vi "Diagnostic Unlock ECU Service.vi"(10 "NIVS.Workspace Event":refnum<event-registration>, 11 "NIVS.Gateway IP Address":string="localhost") -> ()   [LabVIEW 2024, in "Diagnostic Unlock ECU Service.lvlib"]
uses:
  Diagnostic Unlock ECU Service.lvlib
  Types/State Variables.ctl
  <vilib>/NI VeriStand/Execution/Workspace/WorkspaceAPI.ctl
  <vilib>/Platform/TimedLoop/XDataNode/timing_clust.ctl
  <vilib>/Platform/TimedLoop/XDataNode/nitl_modes.ctl
  <vilib>/Platform/TimedLoop/XDataNode/wakeup.ctl
  <vilib>/Utility/error.llb/DialogType.ctl
  <vilib>/Platform/TimedLoop/XDataNode/XDataNode.xnode
  <vilib>/NI VeriStand/Execution/Workspace/NI_VS Workspace ExecutionAPI.lvlib
  <vilib>/Platform/TimedLoop/XDataNode/XDNodeRunTimeDep.lvlib
  <vilib>/Utility/SystemLogging/NI_SystemLogging.lvlib
  NationalInstruments.VeriStand.ClientAPI
panel:
  in  "Stop":bool
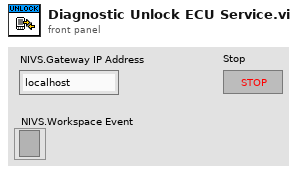
[diagram p1: front panel]
types:
  T1 = typedef "Diagnostic Unlock ECU Service.lvlib/State Variables.ctl" = cluster{"VS.Workspace.Ref":T2, "VS.Connected?":bool, "TCP.Listener":refnum<k5>, "Name":string}
  T2 = typedef "NI_VS Workspace ExecutionAPI.lvlib/WorkspaceAPI.ctl" = refnum<k24>
  T3 = typedef "NI_VS Workspace ExecutionAPI.lvlib/SystemStateEventRef.ctl" = cluster{"CustDatRef":refnum<user-event>, "EvtRef":refnum<k27>, "Target State User Event":refnum<user-event>}
  T4 = typedef "NI_VS Workspace ExecutionAPI.lvlib/SystemStateRegEventRef.ctl" = refnum<event-registration>
  T5 = cluster{"NIVS.Workspace Event":refnum<event-registration>, "SystemChangeEventRef":T4}
  T6 = typedef "XDNodeRunTimeDep.lvlib/timing_clust.ctl" = cluster{"Expected End [f-1]":u64, "Actual End [f-1]":u64, "Finished Late? [f-1]":bool, "Expected End [i-1]":u64, "Actual End [i-1]":u64, "Finished Late? [i-1]":bool, "Expected Start [i]":u64, "Actual Start [i]":u64, "Expected Start [f]":u64, "Actual Start [f]":u64, "Source Name":string, "Structure Name":string, "Period":i64, "Deadline":i64, "Offset":i64, "Start":i64, "Priority":i32, "Timeout":i32, "Mode":T7, "Wakeup Reason":T8, "Error":errorcluster, "Source Type":string, "Secondary Source Type":string, "Global End Time":u64, "Global Start Time":u64, "Frame Duration":u64, "Iteration Duration":u64, "Assigned CPU":i32, "I/O Scan Engine Mode":u32}
  T7 = typedef "XDNodeRunTimeDep.lvlib/nitl_modes.ctl" = enum32{"No Change", "Process missed periods, maintain original phase", "Discard missed periods, maintain original phase", "Process missed periods, ignore original phase", "Discard missed periods, ignore original phase"}
  T8 = typedef "XDNodeRunTimeDep.lvlib/wakeup.ctl" = enum32{"Normal", "Aborted", "Asynchronous wakeup", "Timing source error", "Timed loop error", "Timeout"}
  T9 = typedef "NI_VS Workspace ExecutionAPI.lvlib/SystemState.ctl" = u8
  T10 = typedef "DialogType.ctl" = u16
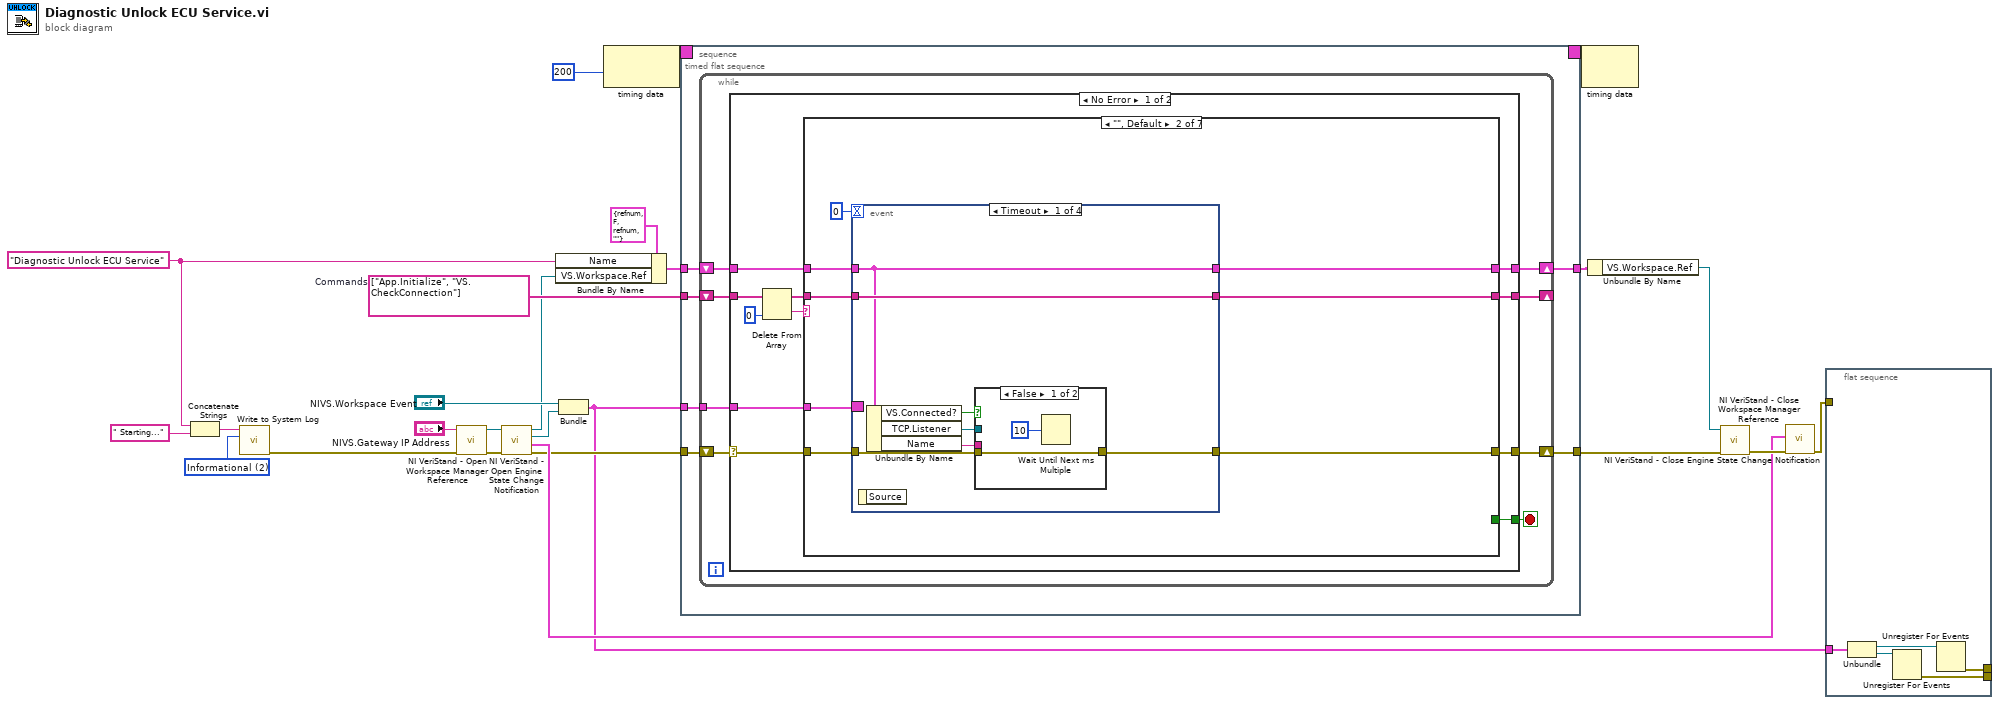
[diagram p0: block diagram]
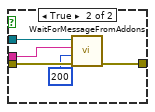
[diagram p3: hidden frame]
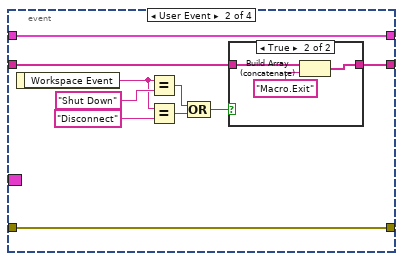
[diagram p4: hidden frame]
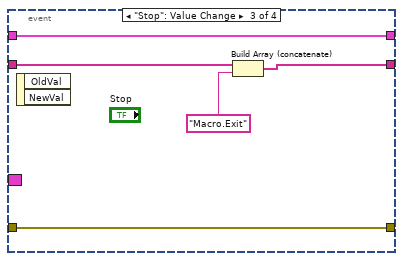
[diagram p6: hidden frame]
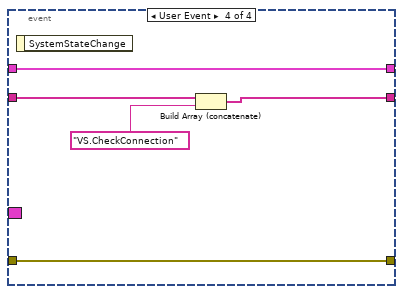
[diagram p7: hidden frame]
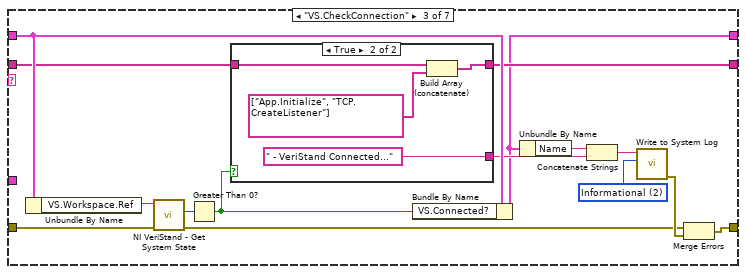
[diagram p8: hidden frame]
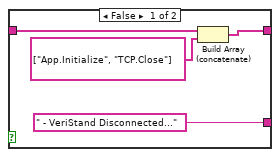
[diagram p9: hidden frame]
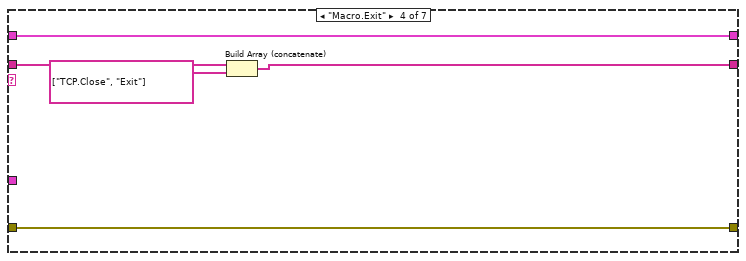
[diagram p10: hidden frame]
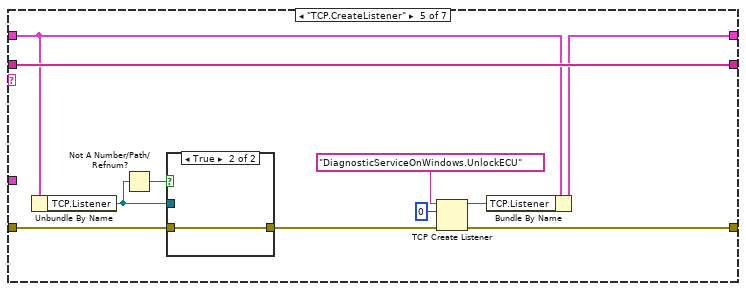
[diagram p11: hidden frame]
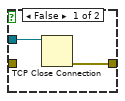
[diagram p12: hidden frame]
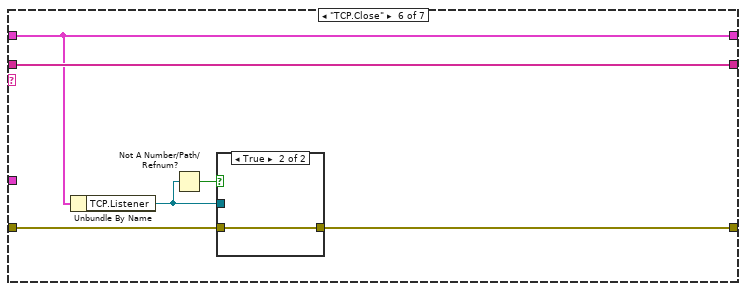
[diagram p13: hidden frame]
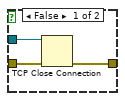
[diagram p14: hidden frame]
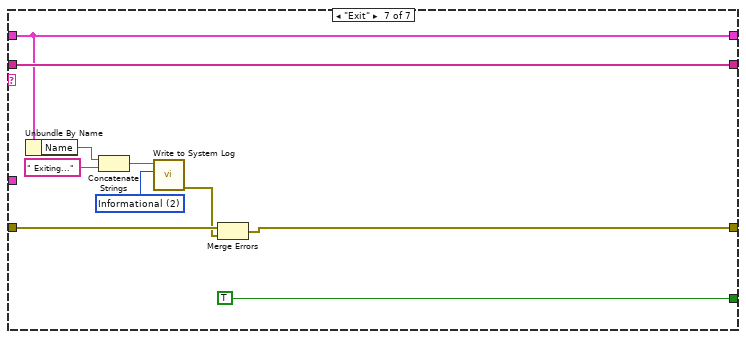
[diagram p15: hidden frame]
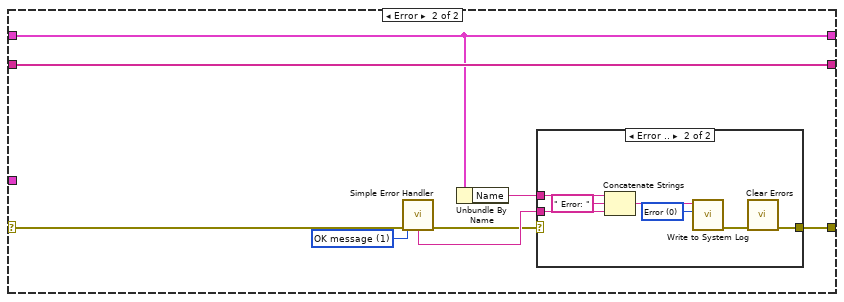
[diagram p16: hidden frame]
diagram:
  w1 = "Diagnostic Unlock ECU Service" ("string")
  w8 = 2 items=["Error", "Warning", "Informational"] ("severity")
  w19 = string[] ["App.Initialize", "VS.CheckConnection"]  # Commands
  n1 = Concatenate Strings(w1, " Starting..." ("message")) -> (w3:string)
  n2 = call <vilib>:"Write to System Log.vi"("severity"=w8, "message"=w3) -> ("error out"=w7:errorcluster)  [unwired: 9 in]
  n3 = call <vilib>:"NI VeriStand - Open Workspace Manager Reference.vi"("error in (no error)"=w7, "Gateway IP Address (\"\": localhost)"="NIVS.Gateway IP Address") -> ("error out"=w5:errorcluster, "WorkspaceManager"=w25:T2)  [unwired: 8 in]
  n4 = call <vilib>:"NI VeriStand - Open Engine State Change Notification.vi"("error in (no error)"=w5, "WorkspaceManager in"=w25) -> ("error out"=w20:errorcluster, "SystemStateRefs"=w23:T3, "SystemChangeEventRef"=w21:T4, "WorkspaceManager out"=w16:T2)  [unwired: 6 in]
  n5 = Bundle By Name(cluster=T1 {"VS.Workspace.Ref"=refnum, "VS.Connected?"=FALSE, "TCP.Listener"=refnum, "Name"=""}, "Name"=w1, "VS.Workspace.Ref"=w16) -> (w14:T1)
  n6 = Bundle("NIVS.Workspace Event"="NIVS.Workspace Event", "SystemChangeEventRef"=w21) -> (w18:T5)  [unwired: 1 in]
  n7 = node-c288(200 ("Priority")) -> (w11:T6)
  n8 = timed-sequence {
    timing: w11 -> [_]
    timing-out: [_] -> w10
    tunnel: [w31] -> w4
    tunnel: w20 -> [w30]
    tunnel: w19 -> [w29]
    tunnel: w18 -> [w28]
    tunnel: w14 -> [w27]
    tunnel: [w26] -> w13
    n9 = timed-flat-sequence {
      tunnel: [w37] -> w31
      tunnel: w30 -> [w36]
      tunnel: w29 -> [w35]
      tunnel: w28 -> [w34]
      tunnel: w27 -> [w33]
      tunnel: [w32] -> w26
      n10 = while {
        tunnel: w34 -> [w45]
        shift-right: [w44] -> w37
        shift-left: w36 -> [w42]
        shift-right: [w39] -> w32
        shift-left: w33 -> [w43]
        shift-right: [w40] -> _
        shift-left: w35 -> [w41]
        stop <- w38 stop-if-true
        n11 = case shown="No Error" w42 {
          selector: w42 -> [w52 w170]
          tunnel: w45 -> [w56 _]
          tunnel: [w55 w172] -> w44
          tunnel: [w54 _] -> w38
          tunnel: w43 -> [w53 w169]
          tunnel: w41 -> [w51 w175]
          tunnel: [w47 w175] -> w40
          tunnel: [w46 w169] -> w39
          frame No Error {
            n12 = Delete From Array(array=w51, index=0) -> (deleted portion=w49:string, array with subset deleted=w48:string[])  [unwired: 1 in]
            n13 = case shown="\"\", Default" w49 {
              tunnel: w56 -> [_ w67 _ _ _ _ _]
              tunnel: w52 -> [w58 w66 w120 w129 w134 w150 w163]
              tunnel: [w58 w65 w108 w129 w143 w151 w161] -> w55
              tunnel: [_ _ _ _ _ _ TRUE] -> w54
              tunnel: w53 -> [w57 w61 w118 w131 w137 w152 w160]
              tunnel: w48 -> [w59 w64 w114 w133 w144 w153 w166]
              tunnel: [w59 w63 w115 w132 w144 w153 w166] -> w47
              tunnel: [w57 w62 w107 w131 w139 w152 w160] -> w46
              frame "App.Initialize" {
              }
              frame "", Default {
                n14 = event shown="[0] Timeout" {
                  selector: w67 -> [_ _ _ _]
                  dyn-events: _ -> [_ _ _ _]
                  timeout: 0 -> [_ _ _ _]
                  tunnel: w66 -> [w70 w91 w100 w105]
                  tunnel: [w71 w91 w100 w105] -> w65
                  tunnel: w61 -> [w73 w90 w99 w101]
                  tunnel: w64 -> [w74 w89 w98 w104]
                  tunnel: [w74 w87 w97 w103] -> w63
                  tunnel: [w73 w90 w99 w101] -> w62
                  event Timeout {
                    n15 = event-data() -> ()  [unwired: 1 in, 1 out]
                    n16 = Unbundle By Name(w73) -> ("VS.Connected?"=w68:bool, "TCP.Listener"=w72:refnum<k5>, "Name"=w69:string)
                    n17 = case shown="False" w68 {
                      tunnel: w72 -> [_ w81]
                      tunnel: [w76 w80] -> w71
                      tunnel: w70 -> [w76 w79]
                      tunnel: w69 -> [_ w78]
                      frame False {
                        n18 = Wait Until Next ms Multiple(millisecond multiple=u32 10 ("Publish.Period_ms")) -> ()  [unwired: 1 out]
                      }
                      frame True {
                        n19 = call "WaitForMessageFromAddons.vi"("error in (no error)"=w79, "timeout ms"=200, "Name"=w78, "TCP Ref"=w81) -> ("error out"=w80:errorcluster)  [unwired: 7 in]
                      }
                    }
                  }
                  event User Event {
                    n20 = event-data() -> ("Workspace Event"=w82:string)  [unwired: 1 in]
                    n21 = Equal?(x=w82, y="Shut Down") -> (x = y?=w84:bool)
                    n22 = Equal?(x=w82, y="Disconnect") -> (x = y?=w85:bool)
                    n23 = Compound Arithmetic op=OR(w84, w85) -> (w83:bool)
                    n24 = case shown="True" w83 {
                      tunnel: w89 -> [w92 w95]
                      tunnel: [w92 w94] -> w87
                      frame False {
                      }
                      frame True {
                        n25 = Build Array (concatenate)(w95, "Macro.Exit" ("y")) -> (w94:string[])
                      }
                    }
                  }
                  event "Stop": Value Change {
                    n26 = event-data() -> ()  [unwired: 1 in, 2 out]
                    n27 = Build Array (concatenate)(w98, "Macro.Exit" ("y")) -> (w97:string[])
                  }
                  event User Event {
                    n28 = event-data() -> ()  [unwired: 1 in, 1 out]
                    n29 = Build Array (concatenate)(w104, "VS.CheckConnection") -> (w103:string[])
                  }
                }
              }
              frame "VS.CheckConnection" {
                w113 = 2 items=["Error", "Warning", "Informational"] ("severity")
                n30 = Unbundle By Name(w118) -> ("VS.Workspace.Ref"=w119:T2)
                n31 = call <vilib>:"NI VeriStand - Get System State.vi"("error in (no error)"=w120, "WorkspaceManager in"=w119) -> ("error out"=w109:errorcluster, "System State"=w117:T9)  [unwired: 5 in, 3 out]
                n32 = Greater Than 0?(x=w117) -> (x > 0?=w116:bool)
                n33 = case shown="True" w116 {
                  tunnel: [w123 w127] -> w115
                  tunnel: w114 -> [w122 w128]
                  tunnel: [" - VeriStand Disconnected..." " - VeriStand Connected..."] -> w112
                  frame False {
                    n34 = Build Array (concatenate)(w122, string[] ["App.Initialize", "TCP.Close"]) -> (w123:string[])
                  }
                  frame True {
                    n35 = Build Array (concatenate)(w128, string[] ["App.Initialize", "TCP.CreateListener"]) -> (w127:string[])
                  }
                }
                n36 = Bundle By Name(cluster=w118, "VS.Connected?"=w116) -> (w107:T1)
                n37 = Unbundle By Name(w107) -> ("Name"=w106:string)
                n38 = Concatenate Strings(w106, w112) -> (w111:string)
                n39 = call <vilib>:"Write to System Log.vi"("severity"=w113, "message"=w111) -> ("error out"=w110:errorcluster)  [unwired: 9 in]
                n40 = Merge Errors(w109, w110) -> (w108:errorcluster)
              }
              frame "Macro.Exit" {
                n41 = Build Array (concatenate)(w133, string[] ["TCP.Close", "Exit"]) -> (w132:string[])
              }
              frame "TCP.CreateListener" {
                n42 = Unbundle By Name(w137) -> ("TCP.Listener"=w136:refnum<k5>)
                n43 = Not A Number/Path/Refnum?(number/path/refnum=w136) -> (NaN/Path/Refnum?=w138:bool)
                n44 = case shown="True" w138 {
                  tunnel: [w146 w147] -> w135
                  tunnel: w136 -> [w145 _]
                  tunnel: w134 -> [_ w147]
                  frame False {
                    n45 = TCP Close Connection(connection ID=w145) -> (error out=w146:errorcluster)  [unwired: 2 in, 1 out]
                  }
                  frame True {
                  }
                }
                n46 = TCP Create Listener(8:w135, 10:u16 0 ("port"), 11:"DiagnosticServiceOnWindows.UnlockECU" ("Host IP Address")) -> (0:w143:errorcluster, 3:w140:refnum<k5>)  [unwired: 2 in, 1 out]
                n47 = Bundle By Name(cluster=w137, "TCP.Listener"=w140) -> (w139:T1)
              }
              frame "TCP.Close" {
                n48 = Unbundle By Name(w152) -> ("TCP.Listener"=w149:refnum<k5>)
                n49 = Not A Number/Path/Refnum?(number/path/refnum=w149) -> (NaN/Path/Refnum?=w148:bool)
                n50 = case shown="True" w148 {
                  tunnel: [w156 w157] -> w151
                  tunnel: w150 -> [w155 w157]
                  tunnel: w149 -> [w154 _]
                  frame False {
                    n51 = TCP Close Connection(connection ID=w154, error in (no error)=w155) -> (error out=w156:errorcluster)  [unwired: 1 in, 1 out]
                  }
                  frame True {
                  }
                }
              }
              frame "Exit" {
                w165 = 2 items=["Error", "Warning", "Informational"] ("severity")
                n52 = Unbundle By Name(w160) -> ("Name"=w158:string)
                n53 = Concatenate Strings(w158, " Exiting..." ("message")) -> (w159:string)
                n54 = call <vilib>:"Write to System Log.vi"("severity"=w165, "message"=w159) -> ("error out"=w162:errorcluster)  [unwired: 9 in]
                n55 = Merge Errors(w163, w162) -> (w161:errorcluster)
              }
            }
          }
          frame Error {
            w174 = T10 1 items=["no dialog", "OK message", "continue or stop message", "OK message + warnings", "continue/stop + warnings"] ("type of dialog (OK msg:1)")
            n56 = call <vilib>:"Simple Error Handler.vi"("type of dialog (OK msg:1)"=w174, "error in (no error)"=w170) -> ("error out"=w171:errorcluster, "message"=w173:string)  [unwired: 3 in, 3 out]
            n57 = Unbundle By Name(w169) -> ("Name"=w168:string)
            n58 = case shown="Error .." w171 {
              selector: w171 -> [w176 _]
              tunnel: w173 -> [_ w177]
              tunnel: [w176 w181] -> w172
              tunnel: w168 -> [_ w180]
              frame No Error {
              }
              frame Error {
                w183 = 0 items=["Error", "Warning", "Informational"] ("severity")
                n59 = Concatenate Strings(w180, " Error: " ("string"), w177) -> (w178:string)
                n60 = call <vilib>:"Write to System Log.vi"("severity"=w183, "message"=w178) -> ("error out"=w182:errorcluster)  [unwired: 9 in]
                n61 = call <vilib>:"Clear Errors.vi"("error in (no error)"=w182) -> ("error out"=w181:errorcluster)  [unwired: 5 in, 1 out]
              }
            }
          }
        }
      }
    }
  }
  n62 = node-c288(w10) -> ()  [unwired: 1 out]
  n63 = Unbundle By Name(w13) -> ("VS.Workspace.Ref"=w12:T2)
  n64 = call <vilib>:"NI VeriStand - Close Workspace Manager Reference.vi"("error in (no error)"=w4, "WorkspaceManager"=w12) -> ("error out"=w24:errorcluster)  [unwired: 9 in]
  n65 = call <vilib>:"NI VeriStand - Close Engine State Change Notification.vi"("error in (no error)"=w24, "SystemStateRefs"=w23) -> ("error out"=w17:errorcluster)  [unwired: 9 in]
  n66 = flat-sequence {
    tunnel: w18 -> [w188]
    tunnel: w17 -> [_]
    tunnel: [w187] -> _
    tunnel: [w186] -> _
    frame #0 {
      n67 = Unbundle(w188) -> ("NIVS.Workspace Event"=w189:refnum<event-registration>, "SystemChangeEventRef"=w190:T4)
      n68 = Unregister For Events(event registration refnum=w190) -> (error out=w186:errorcluster)  [unwired: 1 in]
      n69 = Unregister For Events(event registration refnum=w189) -> (error out=w187:errorcluster)  [unwired: 1 in]
    }
  }
